vi "Emergence stop.vi"(10 "Enable potentiostat":bool, 11 "Configured COM ports":T1={"Pump 1 COM"="COM12", "Pump 2 COM"="COM9", "Pump 3 COM"="COM13", "Pump 4 COM"="COM4", "Pump 5 COM"="COM4"}) -> ()   [LabVIEW 2017]
uses:
  <instrlib>/Harvard Syringe Pump PHD2000/Harvard Syringe Pump PHD2000.lvlib
  <instrlib>/Harvard Apparatus PHD Ultra Series/Harvard Apparatus PHD Ultra Series.lvlib
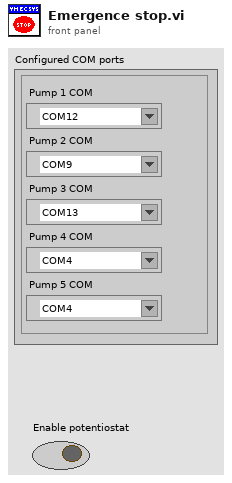
[diagram p1: front panel]
types:
  T1 = cluster{"Pump 1 COM":refnum<visa-resource-name>, "Pump 2 COM":refnum<visa-resource-name>, "Pump 3 COM":refnum<visa-resource-name>, "Pump 4 COM":refnum<visa-resource-name>, "Pump 5 COM":refnum<visa-resource-name>}
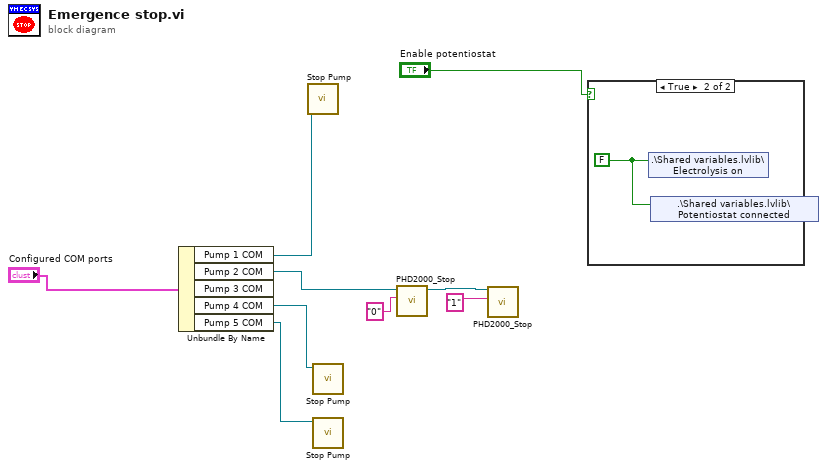
[diagram p0: block diagram]
diagram:
  n1 = Unbundle By Name("Configured COM ports") -> ("Pump 1 COM"=w8:refnum<visa-resource-name>, "Pump 2 COM"=w5:refnum<visa-resource-name>, "Pump 4 COM"=w9:refnum<visa-resource-name>, "Pump 5 COM"=w7:refnum<visa-resource-name>)  [unwired: 1 out]
  n2 = call <instrlib>:"Stop Pump.vi"("VISA resource name"=w8) -> ()  [unwired: 9 in, 2 out]
  n3 = call <instrlib>:"Stop Pump.vi"("VISA resource name"=w9) -> ()  [unwired: 9 in, 2 out]
  n4 = call <instrlib>:"Stop Pump.vi"("VISA resource name"=w7) -> ()  [unwired: 9 in, 2 out]
  n5 = call <instrlib>:"PHD2000_Stop.vi"("VISA resource name 2"=w5, "Pump #"="0") -> ("VISA resource name out"=w2:refnum<visa-resource-name>)  [unwired: 7 in, 1 out]
  n6 = call <instrlib>:"PHD2000_Stop.vi"("VISA resource name 2"=w2, "Pump #"="1") -> ()  [unwired: 7 in, 2 out]
  n7 = case shown="True" "Enable potentiostat" {
    frame False {
    }
    frame True {
      w10 = FALSE ("Electrolysis on")
      n8 = shared-variable ".\\Shared variables.lvlib\\Electrolysis on"(w10) -> ()  [unwired: 1 in, 1 out]
      n9 = shared-variable ".\\Shared variables.lvlib\\Potentiostat connected"(w10) -> ()  [unwired: 1 in, 1 out]
    }
  }
